vi "Get Tx Generic Section.vi"(8 "error in":errorcluster, 11 "Parent section Ref in":T1 format="%.0x") -> (0 "error out":errorcluster, 2 "Item Ref":T1 format="%.0x", 3 "Parent section Ref out":T1 format="%.0x", 4 "Found?":bool)   [LabVIEW 2020, in "AIM ARINC 664 Scripting.lvlib"]
uses:
  AIM ARINC 664 Scripting.lvlib
  <vilib>/NI VeriStand/Custom Device API/Custom Device Item Ref.ctl
  Constants.vi
  <vilib>/NI VeriStand/Custom Device Tools/Custom Device Utility Library/NI VeriStand - Search for Item by GUID.vi
  <vilib>/NI VeriStand/Custom Device Tools/Custom Device Utility Library/Custom Device Utility Library.lvlib
  <vilib>/NI VeriStand/Custom Device API/Custom Device API.lvlib
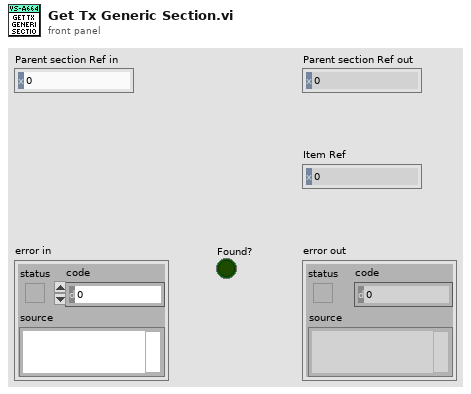
[diagram p1: front panel]
types:
  T1 = typedef "Custom Device API.lvlib/Custom Device Item Ref.ctl" = u64
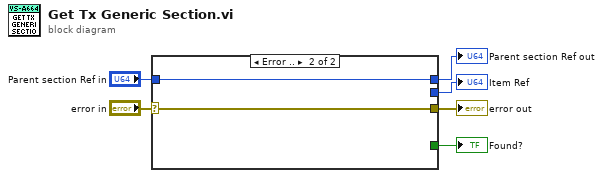
[diagram p0: block diagram]
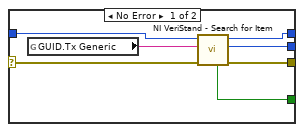
[diagram p2: hidden frame]
diagram:
  n1 = case shown="Error .." "error in" {
    selector: "error in" -> [w8 w14]
    tunnel: "Parent section Ref in" -> [w13 w15]
    tunnel: [w11 _] -> w5
    tunnel: [w10 w15] -> w4
    tunnel: [w9 _] -> w3
    tunnel: [w7 w14] -> w1
    frame No Error {
      n2 = global read "Constants.vi" "GUID.Tx Generic"() -> (w12:string)
      n3 = call-poly <vilib>:"NI VeriStand - Search for Item.vi"("error in"=w8, "Item GUID"=w12, "Section Ref in"=w13) -> ("error out"=w7:errorcluster, "Item Ref"=w9:T1, "Section Ref out"=w10:T1, "Found"=w11:bool)  [unwired: 5 in]
    }
    frame Error {
    }
  }
  "Parent section Ref out" <- w4
  "error out" <- w1
  "Found?" <- w5
  "Item Ref" <- w3
